vi "4.feladat.vi"() -> ()   [LabVIEW 2015]
panel:
  out "csak a for ciklus futási ideje":dbl
  out "átváltás futása":dbl
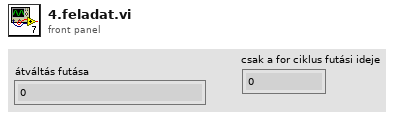
[diagram p1: front panel]
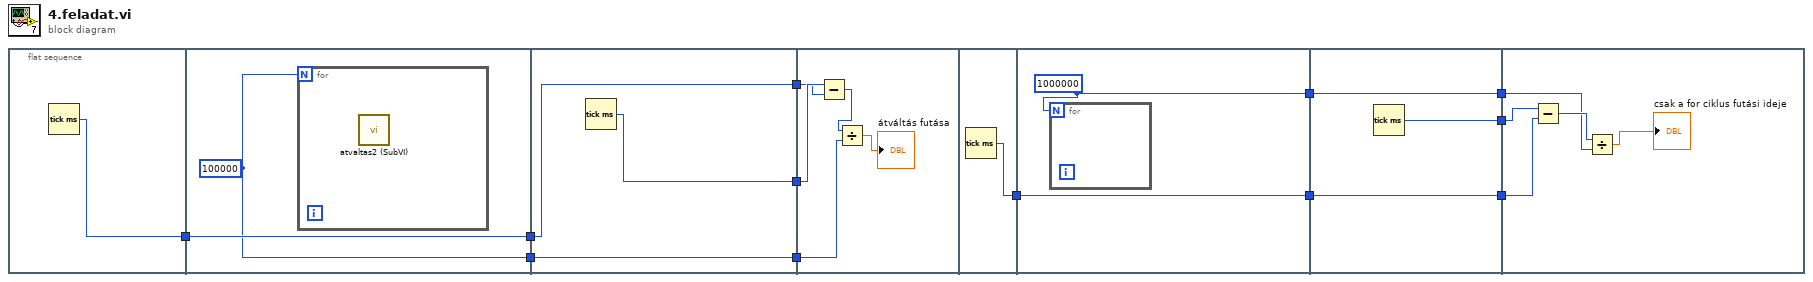
[diagram p0: block diagram]
diagram:
  n1 = flat-sequence {
    tunnel: [w13] -> w11
    tunnel: [w15] -> w12
    tunnel: w11 -> [w15]
    tunnel: [w14] -> w10
    tunnel: w12 -> [w17]
    tunnel: w10 -> [w16]
    tunnel: [w18] -> w9
    tunnel: [w17] -> w8
    tunnel: [w16] -> w7
    tunnel: w9 -> [w20]
    tunnel: w8 -> [w19]
    tunnel: w7 -> [w22]
    tunnel: [w24] -> w4
    tunnel: [w26] -> w5
    tunnel: w4 -> [w26]
    tunnel: [w25] -> w1
    tunnel: [w29] -> w6
    tunnel: w5 -> [w29]
    tunnel: [w28] -> w3
    tunnel: [w27] -> w2
    tunnel: w1 -> [w27]
    tunnel: w6 -> [w30]
    tunnel: w3 -> [w31]
    tunnel: w2 -> [w33]
    frame #0 {
      n2 = Tick Count (ms)() -> (millisecond timer value=w13:u32)
    }
    frame #1 {
      w14 = 100000
      n3 = for {
        N: w14 -> [_]
        n4 = call "atvaltas2 (SubVI).vi"() -> ()  [unwired: 11 in, 1 out]
      }
    }
    frame #2 {
      n5 = Tick Count (ms)() -> (millisecond timer value=w18:u32)
    }
    frame #3 {
      n6 = Subtract(x=w20, y=w19) -> (x-y=w23:u32)
      n7 = Divide(x=w23, y=w22) -> (x/y=→"átváltás futása":dbl)
    }
    frame #4 {
      n8 = Tick Count (ms)() -> (millisecond timer value=w24:u32)
    }
    frame #5 {
      w25 = 1000000
      n9 = for {
        N: w25 -> [_]
      }
    }
    frame #6 {
      n10 = Tick Count (ms)() -> (millisecond timer value=w28:u32)
    }
    frame #7 {
      n11 = Subtract(x=w31, y=w30) -> (x-y=w34:u32)
      n12 = Divide(x=w34, y=w33) -> (x/y=→"csak a for ciklus futási ideje":dbl)
    }
  }
